vi "axex_delete_sheet.vi"(8 "error in":errorcluster, 9 "index of sheet (none)":i32=-1, 10 "sheet name (none)":string, 11 "AX Excel instance in":T1) -> (0 "error out":errorcluster, 3 "AX Excel instance out":T1)   [LabVIEW 2020, in "AX Excel.lvlib"]
doc: "Call this to delete sheet. The sheet to delete can be identified by index or name. If no index nor name is given it deletes current sheet."
uses:
  AX Excel.lvlib
  axex_instance.ctl
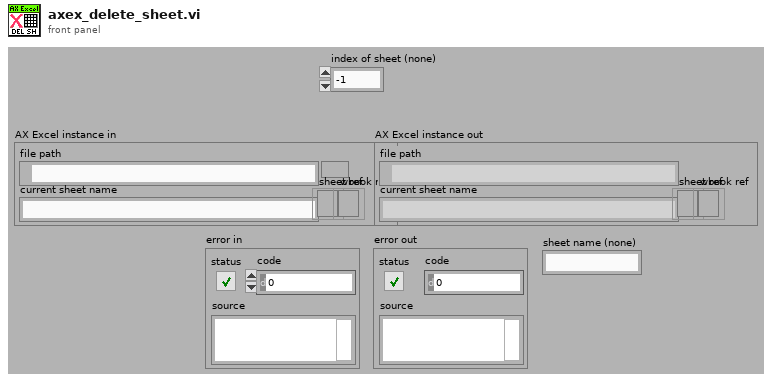
[diagram p1: front panel]
types:
  T1 = typedef "AX Excel.lvlib/axex_instance.ctl" = cluster{"file path":path, "current sheet name":string, "sheet ref":refnum<k7>, "wbook ref":refnum<k7>}
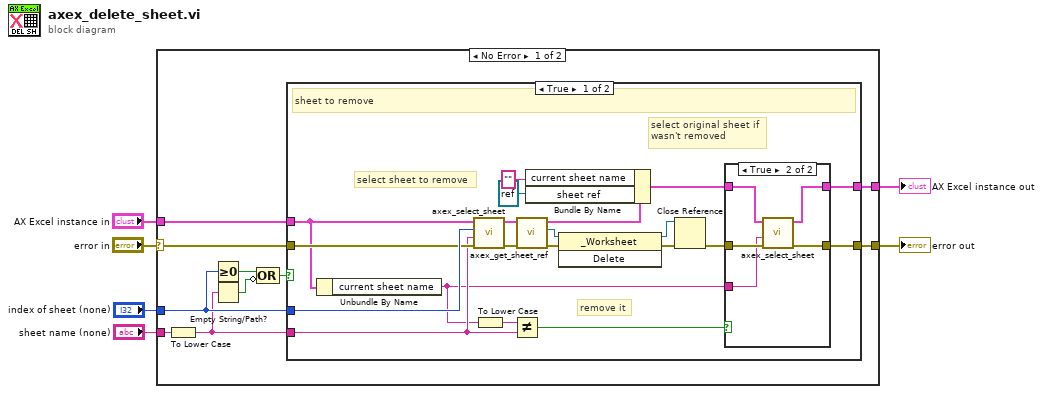
[diagram p0: block diagram]
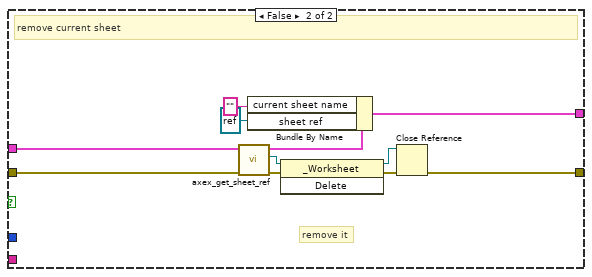
[diagram p3: hidden frame]
diagram:
  n1 = case shown="No Error" "error in" {
    selector: "error in" -> [w7 w56]
    tunnel: "AX Excel instance in" -> [w16 w55]
    tunnel: "index of sheet (none)" -> [w15 _]
    tunnel: "sheet name (none)" -> [w14 _]
    tunnel: [w9 w56] -> w3
    tunnel: [w8 w55] -> w2
    frame No Error {
      n2 = To Lower Case(string=w14) -> (all lower case string=w10:string)
      n3 = Greater Or Equal To 0?(x=w15) -> (x >= 0?=w13:bool)
      n4 = Empty String/Path?(string/path=w10) -> (empty?=w12:bool)
      n5 = Compound Arithmetic op=OR(w13, invert w12) -> (w11:bool)
      n6 = case shown="True" w11 {
        tunnel: w7 -> [w30 w47]
        tunnel: w16 -> [w29 w46]
        tunnel: w10 -> [w24 _]
        tunnel: w15 -> [w36 _]
        tunnel: [w22 w44] -> w9
        tunnel: [w19 w45] -> w8
        frame True {
          # "select original sheet if\nwasn't removed"
          # "remove it"
          # "select sheet to remove"
          # "sheet to remove"
          n7 = Unbundle By Name(w29) -> ("current sheet name"=w18:string)
          n8 = call "axex_select_sheet.vi"("error in"=w30, "sheet name (none)"=w24, "sheet id"=w36, "AX Excel instance in"=w29) -> ("error out"=w35:errorcluster, "AX Excel instance out"=w34:T1)  [unwired: 4 in, 2 out]
          n9 = To Lower Case(string=w18) -> (all lower case string=w25:string)
          n10 = Not Equal?(x=w25, y=w24) -> (x != y?=w21:bool)
          n11 = call "axex_get_sheet_ref.vi"("error in"=w35, "AX Excel instance in"=w34) -> ("error out"=w33:errorcluster, "sheet ref out"=w32:refnum<k7>, "AX Excel instance out"=w31:T1)  [unwired: 6 in, 1 out]
          n12 = Bundle By Name(cluster=w31, "current sheet name"="", "sheet ref"=refnum<k7> refnum) -> (w20:T1)
          n13 = invoke class="_Worksheet" method="Delete"(reference=w32, error in=w33) -> (reference out=w27:refnum<k7>, error out=w28:errorcluster)  [unwired: 1 in, 1 out]
          n14 = Close Reference(reference=w27, error in (no error)=w28) -> (error out=w23:errorcluster)
          n15 = case shown="True" w21 {
            tunnel: w23 -> [w37 w43]
            tunnel: [w37 w42] -> w22
            tunnel: w20 -> [w38 w41]
            tunnel: [w38 w40] -> w19
            tunnel: w18 -> [_ w39]
            frame False {
            }
            frame True {
              n16 = call "axex_select_sheet.vi"("error in"=w43, "sheet name (none)"=w39, "AX Excel instance in"=w41) -> ("error out"=w42:errorcluster, "AX Excel instance out"=w40:T1)  [unwired: 5 in, 2 out]
            }
          }
        }
        frame False {
          # "remove it"
          # "remove current sheet"
          n17 = call "axex_get_sheet_ref.vi"("error in"=w47, "AX Excel instance in"=w46) -> ("error out"=w54:errorcluster, "sheet ref out"=w53:refnum<k7>, "AX Excel instance out"=w52:T1)  [unwired: 6 in, 1 out]
          n18 = Bundle By Name(cluster=w52, "current sheet name"="", "sheet ref"=refnum<k7> refnum) -> (w45:T1)
          n19 = invoke class="_Worksheet" method="Delete"(reference=w53, error in=w54) -> (reference out=w50:refnum<k7>, error out=w51:errorcluster)  [unwired: 1 in, 1 out]
          n20 = Close Reference(reference=w50, error in (no error)=w51) -> (error out=w44:errorcluster)
        }
      }
    }
    frame Error {
    }
  }
  "error out" <- w3
  "AX Excel instance out" <- w2
